vi "DHE_GetDetYSize.vi"() -> (7 "DHE_DetYSize":i32)   [LabVIEW 2016]
uses:
  private/vis/DHE_GBLDriverVariables.vi
panel:
  out "DHE_DetXSize":i32
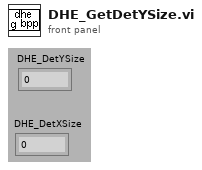
[diagram p1: front panel]
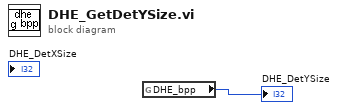
[diagram p0: block diagram]
diagram:
  n1 = global read "DHE_GBLDriverVariables.vi" "DHE_bpp"() -> (→"DHE_DetYSize":i32)
